vi "Autoscale.vi"(8 "error in (no error)":errorcluster, 11 "PXIe5105 in":refnum<class "PXIe5105.lvclass">) -> (0 "error out":errorcluster, 3 "PXIe5105 out":refnum<class "PXIe5105.lvclass">)   [LabVIEW 2018, in "PXIe5105.lvlib" / "PXIe5105.lvclass"]
doc: "This Override method is used to call the Oscope instrument Autoscale function."
uses:
  PXIe5105.lvclass
  PXIe5105.lvclass/PXIe5105.ctl
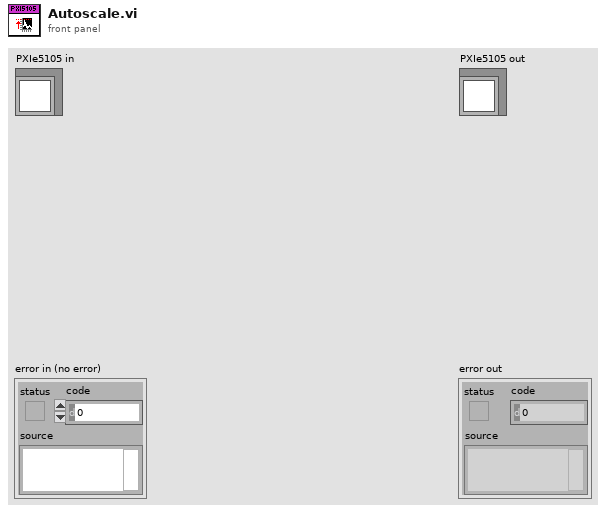
[diagram p1: front panel]
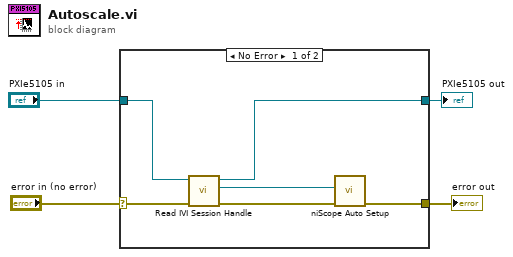
[diagram p0: block diagram]
diagram:
  n1 = case shown="No Error" "error in (no error)" {
    selector: "error in (no error)" -> [w8 w12]
    tunnel: [w10 w12] -> w3
    tunnel: [w7 w11] -> w2
    tunnel: "PXIe5105 in" -> [w9 w11]
    frame No Error {
      n2 = call "Read IVI Session Handle.vi"("error in (no error)"=w8, "PXIe5105 in"=w9) -> ("error out"=w6:errorcluster, "IVI Session Handle"=w5:refnum<k15>, "PXIe5105 out"=w7:refnum<class "PXIe5105.lvclass">)  [unwired: 7 in]
      n3 = call <instrlib>:"niScope Auto Setup.vi"("instrument handle"=w5, "error in"=w6) -> ("error out"=w10:errorcluster)  [unwired: 12 in, 1 out]
    }
    frame Error {
    }
  }
  "error out" <- w3
  "PXIe5105 out" <- w2
